vi "Get Xtal Freq.vi"(8 "error in (no error)":errorcluster, 11 "RTL-SDR in":refnum<class "RTL-SDR.lvclass">) -> (0 "error out":errorcluster, 1 "Tuner Frequency":u32, 2 "RTL Frequency":u32, 3 "RTL-SDR out":refnum<class "RTL-SDR.lvclass">, 4 "function return":i32)   [LabVIEW 2015, in "RTL-SDR.lvclass"]
uses:
  RTL-SDR.lvclass
panel:
  in  "rtl_freq":u32
  in  "tuner_freq":u32
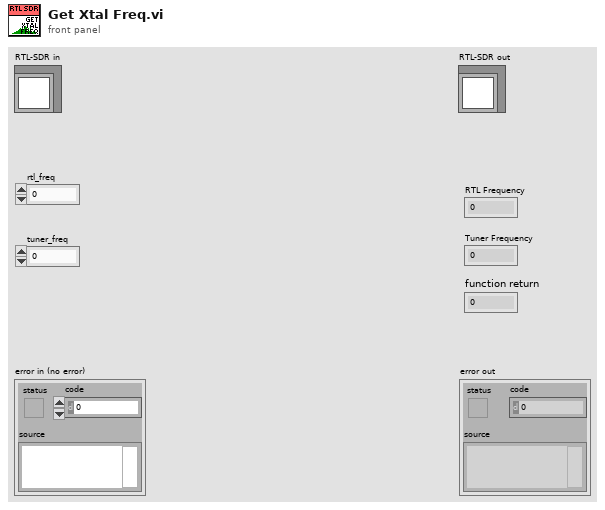
[diagram p1: front panel]
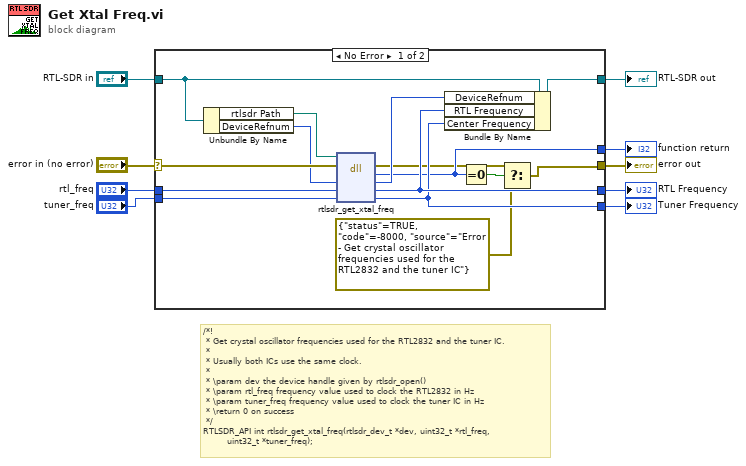
[diagram p0: block diagram]
diagram:
  # "/*!\n * Get crystal oscillator frequencies used for the RTL2832 and the tuner IC.\n *\n * Usually both ICs use the same clock.\n *\n * \\param dev the device handle given by rtlsdr_open()\n * \\param rtl_freq frequency value used to clock the RTL2832 in Hz\n * \\param tuner_freq frequency value used to clock the tuner IC in Hz\n * \\return 0 on success\n */\nRTLSDR_API int rtlsdr_get_xtal_freq(rtlsdr_dev_t *dev, uint32_t *rtl_freq,\n\t\t\t\t    uint32_t *tuner_freq);"
  n1 = case shown="No Error" "error in (no error)" {
    selector: "error in (no error)" -> [w24 w26]
    tunnel: [w10 w26] -> w8
    tunnel: [w22 w25] -> w6
    tunnel: "RTL-SDR in" -> [w23 w25]
    tunnel: "rtl_freq" -> [w18 _]
    tunnel: "tuner_freq" -> [w17 _]
    tunnel: [w12 _] -> w3
    tunnel: [w16 _] -> w2
    tunnel: [w15 _] -> w1
    frame No Error {
      n2 = Unbundle By Name(w23) -> ("rtlsdr Path"=w21:path, "DeviceRefnum"=w20:u64)
      n3 = dll-call lib="C:/Users/Ivan/Desktop/D-23-09-24 (RTL-SDR)/Project (Pelleng-SDR)/RTL-SDR Class/dll/rtlsdr.*" fn="rtlsdr_get_xtal_freq"(path in=w21, error in=w24, "DeviceRefnum"=w20, "rtl_freq"=w18, "tuner_freq"=w17) -> (error out=w11:errorcluster, "return type"=w12:i32, "DeviceRefnum"=w19:u64, "rtl_freq"=w16:u32, "tuner_freq"=w15:u32)  [unwired: 1 in, 1 out]
      n4 = Bundle By Name(cluster=w23, "DeviceRefnum"=w19, "RTL Frequency"=w16, "Center Frequency"=w15) -> (w22:refnum<class "RTL-SDR.lvclass">)
      n5 = Equal To 0?(x=w12) -> (x = 0?=w13:bool)
      n6 = Select(t=w11, s=w13, f=errorcluster {"status"=TRUE, "code"=-8000, "source"="Error - Get crystal oscillator frequencies used for the RTL2832 and the tuner IC"} ("error out")) -> (s? t:f=w10:errorcluster)
    }
    frame Error {
    }
  }
  "error out" <- w8
  "RTL-SDR out" <- w6
  "RTL Frequency" <- w2
  "Tuner Frequency" <- w1
  "function return" <- w3
